vi "FunctionGenerator.vi"() -> ()   [LabVIEW 2015]
doc: "This example demonstrates how to continuously re-generate analog output data from a buffer in your computer's memory.\n\nFor instructions on how to connect your signals to VirtualBench, refer to your hardware documentation."
uses:
  <vilib>/Utility/error.llb/DialogType.ctl
  <vilib>/VirtualBench/_FGEN Configure Standard Waveform4.vi
  <vilib>/VirtualBench/_MSO Configure Analog Channel0.vi
  <vilib>/VirtualBench/_MSO Configure Analog Edge Trigger1.vi
  <vilib>/VirtualBench/_FGEN Configure Standard Waveform29.vi
  <vilib>/VirtualBench/VirtualBench.lvlib
panel:
  out "Trigger Reason":i32(ring) items=["Normal", "Forced", "Auto"]
  in  "Trigger Level":dbl caption="Trigger Level (no change)"
  in  "Stop":bool
  in  "Analog Channel":tag="mso/1" caption="Channel"
  in  "End Frequency (Hz)":dbl=2000000.0 caption="Frequency (no change)" format="%#_6p"
  in  "Number of Steps":i32=200
  in  "Amplitude (V)":dbl=5.0 caption="Amplitude (no change)"
  in  "Start Frequency (Hz)":dbl=500000.0 caption="Frequency (no change)" format="%#_6p"
  in  "DC Offset (V)":dbl caption="DC Offset (no change)"
  in  "VirtualBench Device":tag="VB8012"
  out "Analog Data":waveform(dbl)[](graph)
  # "MSO Channel Settings"
  # "Sine Wave Sweep Settings"
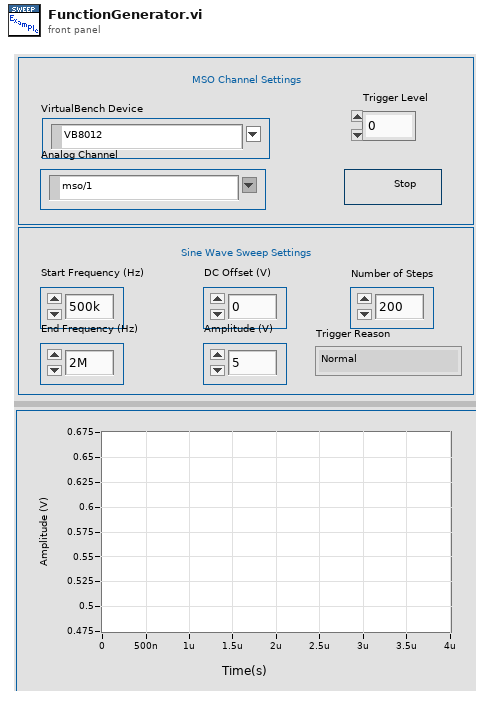
[diagram p1: front panel]
types:
  T1 = typedef "DialogType.ctl" = u16
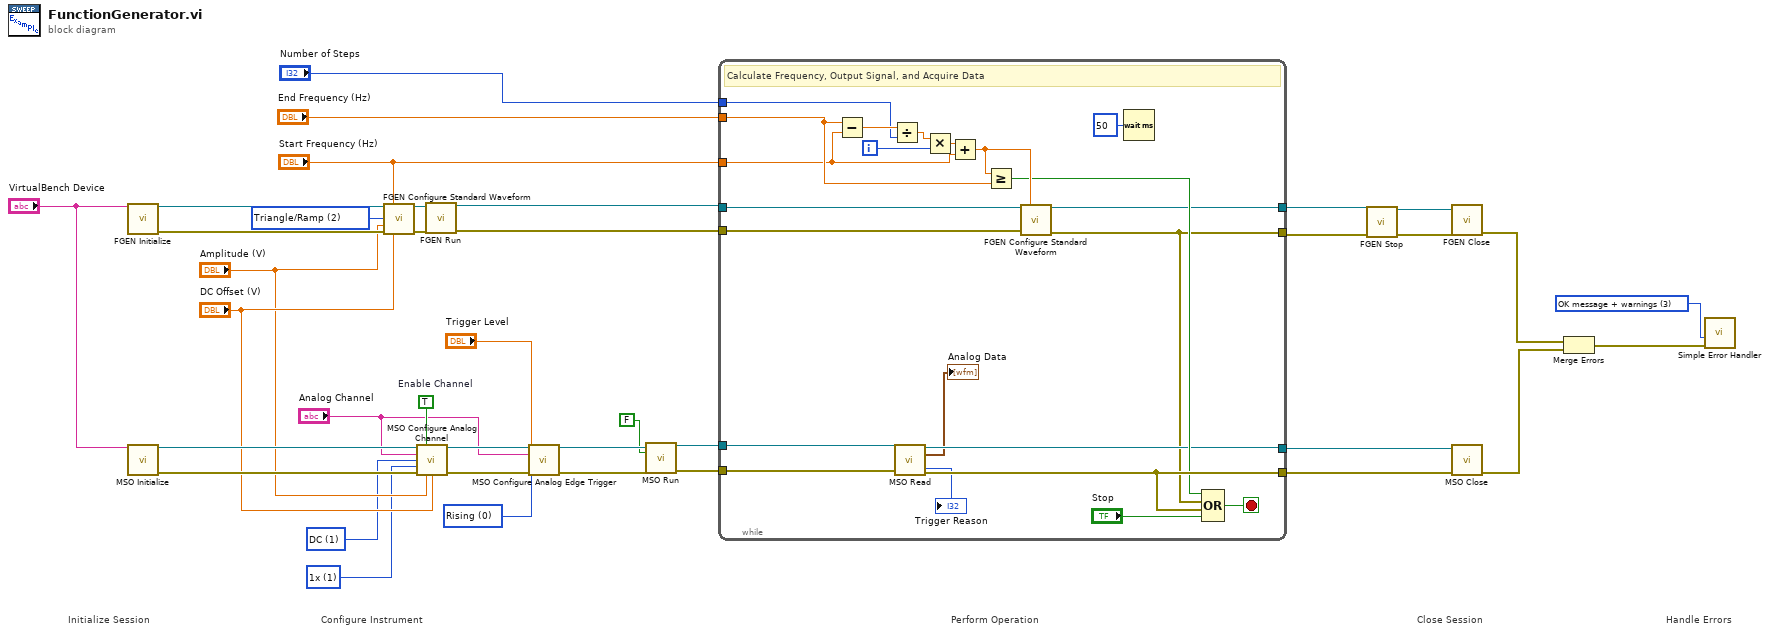
[diagram p0: block diagram]
diagram:
  w7 = 1 items=["1x"=1, "10x"=10] ("Probe Attenuation")
  w8 = 1 items=["AC", "DC"] ("Vertical Coupling")
  w30 = 2 items=["Sine", "Square", "Triangle/Ramp", "DC"] ("Waveform Function")
  w15 = 0 items=["Rising", "Falling", "Either"] ("Trigger Slope")
  w35 = TRUE  # Enable Channel
  w38 = T1 3 items=["no dialog", "OK message", "continue or stop message", "OK message + warnings", "continue/stop + warnings"] ("type of dialog (OK msg:1)")
  # "Handle Errors"
  # "Close Session"
  # "Perform Operation"
  # "Configure Instrument"
  # "Initialize Session"
  n1 = call <vilib>:"FGEN Initialize.vi"("Device Name"="VirtualBench Device") -> ("Instrument Handle Out"=w29:refnum<k21>, "Error Out"=w31:errorcluster)  [unwired: 13 in]
  n2 = call <vilib>:"MSO Initialize.vi"("Device Name"="VirtualBench Device") -> ("Instrument Handle Out"=w33:refnum<k21>, "Error Out"=w34:errorcluster)  [unwired: 13 in]
  n3 = call-poly <vilib>:"FGEN Configure Standard Waveform.vi"("Instrument Handle In"=w29, "Frequency"="Start Frequency (Hz)", "Waveform Function"=w30, "Amplitude"="Amplitude (V)", "Error In"=w31, "DC Offset"="DC Offset (V)") -> ("Instrument Handle Out"=w18:refnum<k21>, "Error Out"=w17:errorcluster)  [unwired: 8 in]
  n4 = call-poly <vilib>:"MSO Configure Analog Channel.vi"("Instrument Handle In"=w33, "Enable Channel"=w35, "Channel"="Analog Channel", "Vertical Coupling"=w8, "Probe Attenuation"=w7, "Error In"=w34, "Vertical Range"="Amplitude (V)", "Vertical Offset"="DC Offset (V)") -> ("Instrument Handle Out"=w25:refnum<k21>, "Error Out"=w24:errorcluster)  [unwired: 6 in]
  n5 = call <vilib>:"FGEN Run.vi"("Instrument Handle In"=w18, "Error In"=w17) -> ("Instrument Handle Out"=w19:refnum<k21>, "Error Out"=w20:errorcluster)  [unwired: 12 in]
  n6 = call-poly <vilib>:"MSO Configure Analog Edge Trigger.vi"("Instrument Handle In"=w25, "Trigger Source"="Analog Channel", "Trigger Slope"=w15, "Trigger Level"="Trigger Level", "Error In"=w24) -> ("Instrument Handle Out"=w5:refnum<k21>, "Error Out"=w3:errorcluster)  [unwired: 9 in]
  n7 = call <vilib>:"MSO Run.vi"("Instrument Handle In"=w5, "Auto Trigger"=FALSE, "Error In"=w3) -> ("Instrument Handle Out"=w4:refnum<k21>, "Error Out"=w2:errorcluster)  [unwired: 11 in]
  n8 = while {
    tunnel: w19 -> [w60]
    tunnel: w20 -> [w54]
    tunnel: "Start Frequency (Hz)" -> [w47]
    tunnel: "End Frequency (Hz)" -> [w50]
    tunnel: [w44] -> w10
    tunnel: [w45] -> w12
    tunnel: "Number of Steps" -> [w58]
    tunnel: [w53] -> w27
    tunnel: [w46] -> w26
    tunnel: w4 -> [w40]
    tunnel: w2 -> [w39]
    i -> [w56]
    stop <- w52 stop-if-true
    # "Calculate Frequency, Output Signal, and Acquire Data"
    n9 = Subtract(x=w50, y=w47) -> (x-y=w59:dbl)
    n10 = Divide(x=w59, y=w58) -> (x/y=w57:dbl)
    n11 = call <vilib>:"MSO Read.vi"("Instrument Handle In"=w40, "Error In"=w39) -> ("Instrument Handle Out"=w46:refnum<k21>, "Analog Waveforms"=→"Analog Data":waveform(dbl)[], "Trigger Reason"=→"Trigger Reason":i32, "Error Out"=w53:errorcluster)  [unwired: 8 in, 2 out]
    n12 = Multiply(x=w57, y=w56) -> (x*y=w55:dbl)
    n13 = Add(x=w55, y=w47) -> (x+y=w51:dbl)
    n14 = Greater Or Equal?(x=w51, y=w50) -> (x >= y?=w49:bool)
    n15 = call-poly <vilib>:"FGEN Configure Standard Waveform.vi"("Instrument Handle In"=w60, "Frequency"=w51, "Error In"=w54) -> ("Instrument Handle Out"=w45:refnum<k21>, "Error Out"=w44:errorcluster)  [unwired: 11 in]
    n16 = Wait (ms)(milliseconds to wait=u32 50) -> ()  [unwired: 1 out]
    n17 = Compound Arithmetic op=OR(w49, w44, w53, "Stop") -> (w52:bool)
  }
  n18 = call <vilib>:"FGEN Stop.vi"("Instrument Handle In"=w12, "Error In"=w10) -> ("Instrument Handle Out"=w11:refnum<k21>, "Error Out"=w9:errorcluster)  [unwired: 12 in]
  n19 = call <vilib>:"FGEN Close.vi"("Instrument Handle In"=w11, "Error In"=w9) -> ("Error Out"=w23:errorcluster)  [unwired: 13 in]
  n20 = call <vilib>:"MSO Close.vi"("Instrument Handle In"=w26, "Error In"=w27) -> ("Error Out"=w22:errorcluster)  [unwired: 13 in]
  n21 = Merge Errors(w23, w22) -> (w21:errorcluster)
  n22 = call <vilib>:"Simple Error Handler.vi"("type of dialog (OK msg:1)"=w38, "error in (no error)"=w21) -> ()  [unwired: 3 in, 5 out]
